vi "Typecast Refnum to Queue.vi"(11 "refnum in":T2) -> (3 "queue out":T1)   [LabVIEW 2020, in "NI_LVConfig.lvlib"]
uses:
  NI_LVConfig.lvlib
  Config Data RefNum.ctl
  <vilib>/Utility/config.llb/Config Queue.ctl
  <vilib>/Utility/config.llb/Config Data.ctl
  Section.ctl
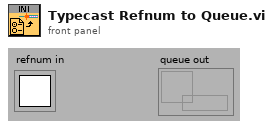
[diagram p1: front panel]
types:
  T1 = typedef "NI_LVConfig.lvlib/Config Queue.ctl" = refnum<queue>
  T2 = typedef "NI_LVConfig.lvlib/Config Data RefNum.ctl" = refnum<k1>
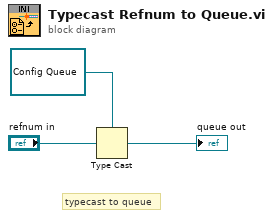
[diagram p0: block diagram]
diagram:
  # "typecast to queue"
  n1 = Type Cast(type=T1 refnum ("queue out"), x="refnum in") -> (*(type *) &x=→"queue out":T1)
